vi "20T_Set_Non_Persistent.vi"(8 "error in (no error)":errorcluster, 11 "Mercury Reference In":T1) -> (0 "error out":errorcluster)   [LabVIEW 2019]
uses:
  Equipment/Mercury iXX/Mercury iXX.lvlib
  Global/Global Variables/Data_Display_global.vi
  Equipment/Mercury iXX/Public/Libraries/Magnet/Open/Open Magnet Device.vi
  Equipment/Mercury iXX/Public/Libraries/Magnet.lvlib
  Equipment/Mercury iXX/Public/Controls/Comms Transport Layer.ctl
  Equipment/Mercury iXX/Private/Controls/Query Dynamic Reference.ctl
  Equipment/Mercury iXX/Public/Controls/Mercury Reference.ctl
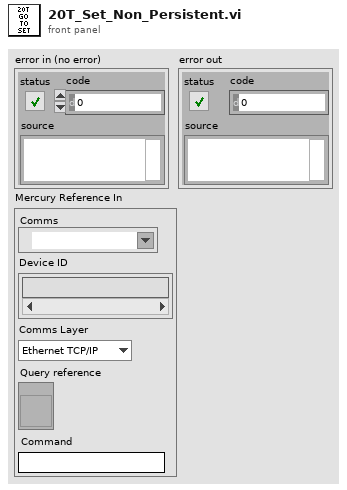
[diagram p1: front panel]
types:
  T1 = typedef "Mercury iXX.lvlib/Mercury Reference.ctl" = cluster{"Comms":refnum<visa-resource-name>, "Device ID":string[], "Comms Layer":T2, "Command":string, "Query reference":T3}
  T2 = typedef "Mercury iXX.lvlib/Comms Transport Layer.ctl" = enum16{"Ethernet TCP/IP", "USB", "ISOBus - RS-232", "GPIB"}
  T3 = typedef "Mercury iXX.lvlib/Query Dynamic Reference.ctl" = refnum<vi>
  T4 = typedef "20T_Cluster.ctl" = cluster{"Clamp":bool, "Switch Heater":bool, "Go to Zero":bool, "Go to set":bool, "Go to Hold":bool, "Clamped":bool, "Quenched":bool, "Rate limit":bool, "Persistent":bool, "Hold":bool, "Set":bool, "Zero":bool, "Magnet (T)":dbl, "Leads (T)":dbl, "Magnet T (K)":dbl, "Switch":bool, "Target (T)":dbl, "Setpoint (T)":dbl, "Rate (T/min)":dbl, "Set Persistent":bool, "Set Rate":bool}
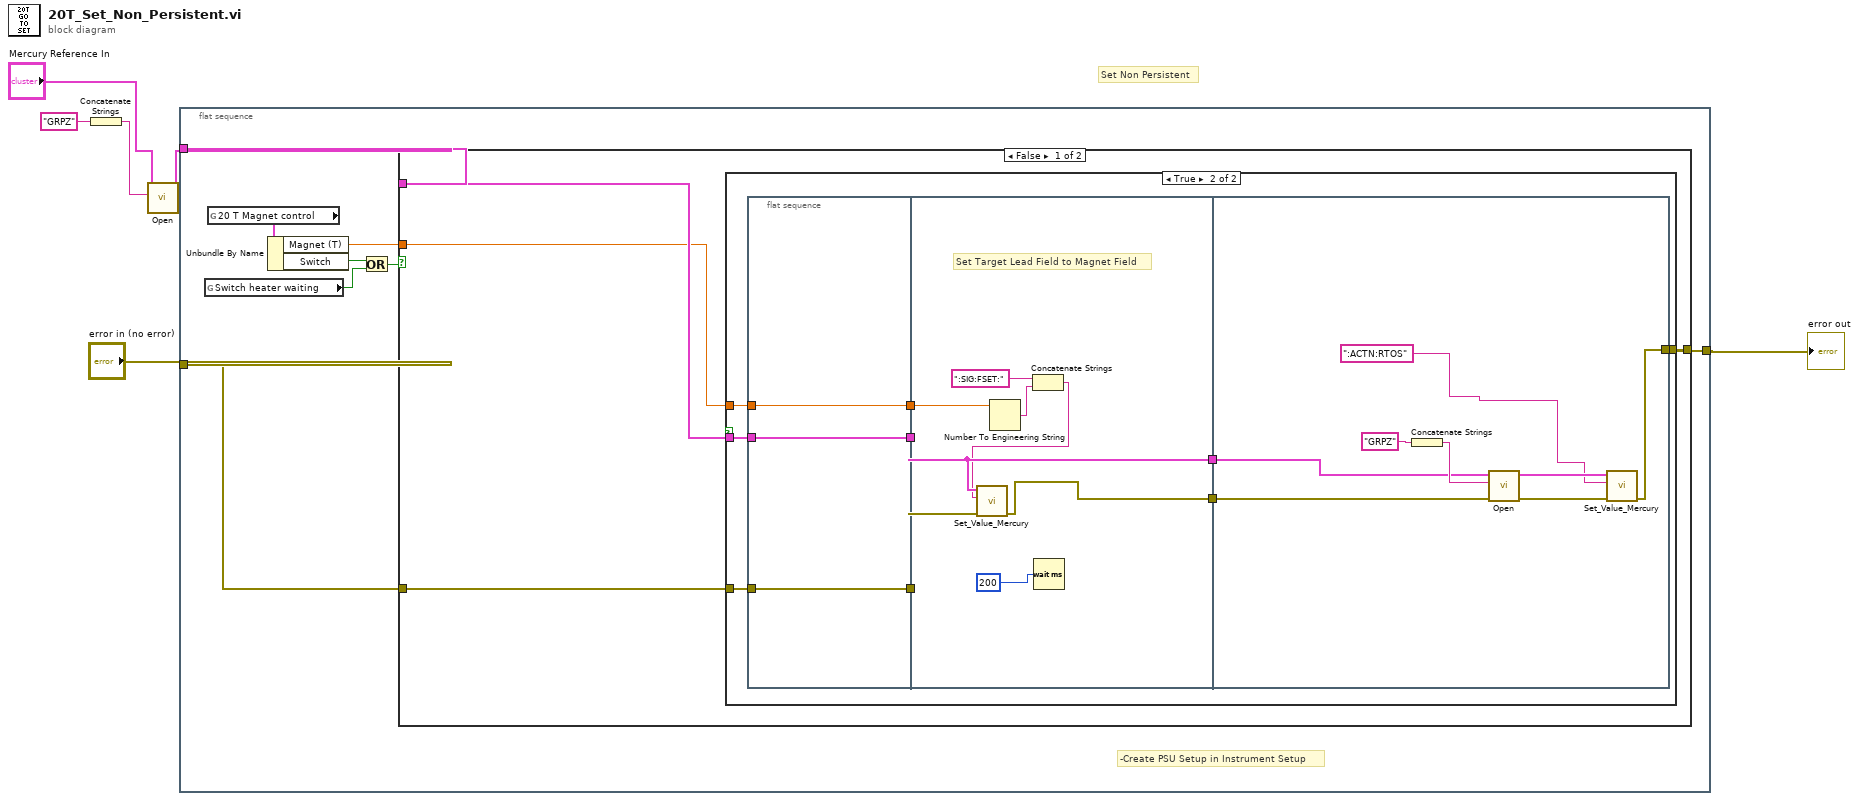
[diagram p0: block diagram]
diagram:
  # "Set Non Persistent"
  n1 = Concatenate Strings("GRPZ" ("Device Identifier")) -> (w5:string)
  n2 = call-poly "Open.vi"("Device Identifier"=w5, "Mercury Reference In"="Mercury Reference In") -> ("Mercury Reference Out"=w2:T1)  [unwired: 2 in, 7 out]
  n3 = flat-sequence {
    tunnel: w2 -> [w11]
    tunnel: "error in (no error)" -> [w9]
    tunnel: [w10] -> w3
    frame #0 {
      # "-Create PSU Setup in Instrument Setup"
      n4 = global read "Data_Display_global.vi" "Switch heater waiting"() -> (w13:bool)
      n5 = global read "Data_Display_global.vi" "20 T Magnet control"() -> (w14:T4)
      n6 = Unbundle By Name(w14) -> ("Magnet (T)"=w7:dbl, "Switch"=w8:bool)
      n7 = Or(x=w8, y=w13) -> (x .or. y?=w12:bool)
      n8 = case shown="False" w12 {
        tunnel: w9 -> [w18 w47]
        tunnel: [w15 w47] -> w10
        tunnel: w11 -> [w17 _]
        tunnel: w7 -> [w16 _]
        frame False {
          n9 = case shown="True" {
            selector: _ -> [_ _]
            tunnel: w18 -> [_ w22]
            tunnel: w17 -> [_ w21]
            tunnel: w16 -> [_ w20]
            tunnel: [_ w19] -> w15
            frame False {
            }
            frame True {
              n10 = flat-sequence {
                tunnel: w20 -> [w28]
                tunnel: w22 -> [w29]
                tunnel: w21 -> [w30]
                tunnel: [w30] -> w27
                tunnel: [w29] -> w26
                tunnel: [w28] -> w25
                tunnel: [w34] -> w24
                tunnel: [w32] -> w23
                tunnel: w27 -> [w32]
                tunnel: w26 -> [w33]
                tunnel: w25 -> [w35]
                tunnel: w24 -> [w41]
                tunnel: w23 -> [w40]
                tunnel: [w39] -> w19
                frame #0 {
                }
                frame #1 {
                  # "Set Target Lead Field to Magnet Field"
                  n11 = Number To Engineering String(4:w35) -> (0:w38:string)  [unwired: 3 in]
                  n12 = Concatenate Strings(":SIG:FSET:", w38) -> (w31:string)
                  n13 = call "Set_Value_Mercury.vi"("error in"=w33, "Noun(s)"=w31, "Mercury Reference In"=w32) -> ("error out"=w34:errorcluster)  [unwired: 7 in, 1 out]
                  n14 = Wait (ms)(milliseconds to wait=200) -> ()  [unwired: 1 out]
                }
                frame #2 {
                  n15 = Concatenate Strings("GRPZ" ("Device Identifier")) -> (w46:string)
                  n16 = call-poly "Open.vi"("error in (no error)"=w41, "Device Identifier"=w46, "Mercury Reference In"=w40) -> ("error out"=w42:errorcluster, "Mercury Reference Out"=w44:T1)  [unwired: 1 in, 6 out]
                  n17 = call "Set_Value_Mercury.vi"("error in"=w42, "Noun(s)"=":ACTN:RTOS", "Mercury Reference In"=w44) -> ("error out"=w39:errorcluster)  [unwired: 7 in, 1 out]
                }
              }
            }
          }
        }
        frame True {
        }
      }
    }
  }
  "error out" <- w3
